vi "Reset.vi"(0 "VISA resource name":refnum<visa-resource-name>, 11 "error in (no error)":errorcluster) -> (4 "VISA resource name out":refnum<visa-resource-name>, 15 "error out":errorcluster)   [LabVIEW 2016, in "APT 300XAC Series.lvlib"]
doc: "Reset the instrument to <B>original power on configuration</B>. Does not clear Enable register for Standard Summary Status or Standard Event Registers. Does not clear the output queue. Does not clear the power-on-status-clear flag."
uses:
  APT 300XAC Series.lvlib
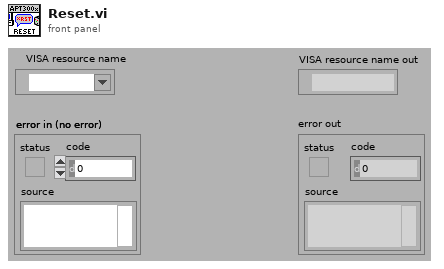
[diagram p1: front panel]
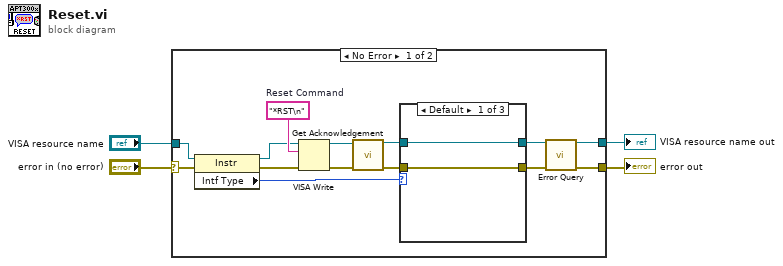
[diagram p0: block diagram]
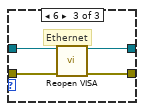
[diagram p3: hidden frame]
diagram:
  n1 = case shown="No Error" "error in (no error)" {
    selector: "error in (no error)" -> [w13 w27]
    tunnel: "VISA resource name" -> [w12 w28]
    tunnel: [w18 w28] -> w3
    tunnel: [w17 w27] -> w2
    frame No Error {
      w16 = "*RST\n"  # Reset Command
      n2 = property on="Property Node" class="Instr"(reference=w12, error in=w13) -> (reference out=w11:refnum<visa-resource-name>, error out=w10:errorcluster, "Intf Type"=w9:u16)
      n3 = VISA Write(VISA resource name=w11, write buffer=w16, error in (no error)=w10) -> (VISA resource name out=w14:refnum<visa-resource-name>, error out=w15:errorcluster)  [unwired: 1 out]
      n4 = call "Get Acknowledgement.vi"("VISA resource name"=w14, "error in (no error)"=w15) -> ("VISA resource name out"=w6:refnum<visa-resource-name>, "error out"=w8:errorcluster)  [unwired: 12 in]
      n5 = case shown="Default" w9 {
        tunnel: w8 -> [w20 w22 w25]
        tunnel: [w20 w22 w24] -> w7
        tunnel: w6 -> [w19 w21 w26]
        tunnel: [w19 w21 w23] -> w5
        frame Default {
        }
        frame 1, 4 {
          # "GPIB. Serial"
        }
        frame 6 {
          # "Ethernet"
          n6 = call "Reopen VISA.vi"("VISA resource name"=w26, "error in (no error)"=w25) -> ("VISA resource name out"=w23:refnum<visa-resource-name>, "error out"=w24:errorcluster)  [unwired: 12 in]
        }
      }
      n7 = call "Error Query.vi"("VISA resource name"=w5, "error in (no error)"=w7) -> ("VISA resource name out"=w18:refnum<visa-resource-name>, "error out"=w17:errorcluster)  [unwired: 10 in, 2 out]
    }
    frame Error {
    }
  }
  "error out" <- w2
  "VISA resource name out" <- w3
